vi "Update-GUI-default-params.vi"(8 "error in":errorcluster, 10 "Data ref. in":refnum<data-value>, 11 "UI ref. in":refnum<data-value>) -> (0 "error IO":errorcluster, 2 "Data ref.":refnum<data-value>, 3 "UI ref.":refnum<data-value>)   [LabVIEW 2013, in "CameraVision.lvlib" / "CV-UI.lvclass"]
doc: "This function loads the default values for the GUI program parameters from an .xml file and writes these values to the GUI controls.\nThe file path for the GUI parameters is '<Application directory>\\Program data\\parameters-gui.xml'.\nThe default hidden parameters can be changed using the 'CV-Set-gui-parameters.vi' utility."
uses:
  CV-UI.lvclass
  Main/CV-Main.lvclass
  Parameters-gui.ctl
  Main/Configuration/Configuration-parameters-gui.ctl
  Main/Acquisition/Acquisition-parameters-gui.ctl
  Main/Acquisition/Trigger-modes.ctl
  Main/Acquisition/Exposure-modes.ctl
  Main/Storage/Storage-parameters-gui.ctl
  Main/Storage/Storage-types.ctl
  Main/Correction/Correction-parameters-gui.ctl
  Main/Correction/Smoothing.ctl
  Main/Correction/Background-correction.ctl
  Main/Analysis/Analysis-parameters-gui.ctl
  Main/Temperature/Temperature-parameters-gui.ctl
  Main/Mapping/Mapping-parameters-gui.ctl
  Main/Mapping/Mapping-characteristic.ctl
  Main/Filter/Filter-parameters-gui.ctl
  Main/Filter/Filter-settings.ctl
  Main/Filter/Filter-characteristic.ctl
  Main/Filter/Filter-apply.ctl
  CV-UI.lvclass/CV-UI.ctl
  Read Parameter refs.vi
  <vilib>/Utility/xml.llb/Read From XML File(string).vi
  Main/Filter/CV-Filter.lvclass
  Main/Mapping/CV-Mapping.lvclass
  Main/Temperature/CV-Temperature.lvclass
  Main/Analysis/CV-Analysis.lvclass
  Main/Correction/CV-Correction.lvclass
  Main/Storage/CV-Storage.lvclass
  Main/Acquisition/CV-Acquisition.lvclass
  Main/Configuration/CV-Configuration.lvclass
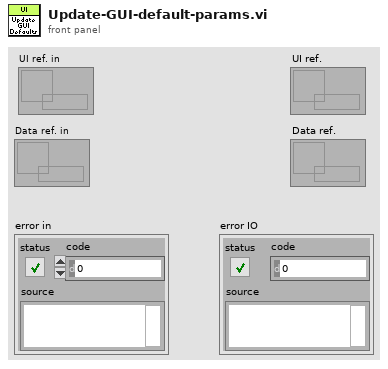
[diagram p1: front panel]
types:
  T1 = typedef "CameraVision.lvlib/CV-UI.lvclass/Parameters-gui.ctl" = cluster{"Configuration params":T2, "Acquisition params":T3, "Storage params":T6, "Correction params":T8, "Analysis params":T11, "Temperature params":T12, "Mapping params":T13, "Filter params":T15}
  T2 = typedef "CameraVision.lvlib/CV-Configuration.lvclass/Configuration-parameters-gui.ctl" = cluster{"Number of cameras":i32, "Camera 1 port":enum16{"A", "B"}, "ROI width":u32, "ROI height":u32, "Reset ROI":bool, "Width scale":dbl, "Height scale":dbl, "Center Y cam. 1":i32, "Center X cam. 1":i32, "Center Y cam. 2":i32, "Center X cam. 2":i32}
  T3 = typedef "CameraVision.lvlib/CV-Acquisition.lvclass/Acquisition-parameters-gui.ctl" = cluster{"Acquisition mode":enum16{"Continuous", "Continuous batch", "Single batch", "Single batch -delayed"}, "Batch size":i32, "Image buffer size":i32, "Trigger mode":T4, "Duration HH":sgl, "Acquisition start":enum16{"Immediate", "Post-phoned"}, "Duration SS":sgl, "Duration MM":sgl, "Start time":timestamp, "Max. frame rate":dbl, "Exposure time cam. 1":dbl, "Exposure time cam. 2":dbl, "Exposure mode":T5, "Value 1":dbl, "Value 2":dbl, "Time 1":dbl, "Time 2":dbl}
  T4 = typedef "CameraVision.lvlib/CV-Acquisition.lvclass/Trigger-modes.ctl" = enum16{"Camera timed (not sync.)", "Framegrabber timed (sync.)", "Software timed (sync.)", "External timing (sync.)", "Manual (sync.)", "Gated - camera (not sync.)", "Gated - grabber (sync.)", "Gated - software (sync.)", "Gated - external (sync.)"}
  T5 = typedef "CameraVision.lvlib/CV-Acquisition.lvclass/Exposure-modes.ctl" = enum16{"Linear", "LinLog"}
  T6 = typedef "CameraVision.lvlib/CV-Storage.lvclass/Storage-parameters-gui.ctl" = cluster{"Base file name":string, "Storage directory":path, "Save what?":T7, "Image file type":enum16{"JPG", "BMP", "PNG"}, "Comments":string, "Storage mode":enum16{"1 file per layer", "1 file for all layers "}, "Start iteration/layer":u16}
  T7 = typedef "CameraVision.lvlib/CV-Storage.lvclass/Storage-types.ctl" = cluster{"Original":bool, "Corrected":bool, "Binary":bool, "Temperature":bool, "Characteristics":bool, "Mapping":bool, "TemperatureValues":bool}
  T8 = typedef "CameraVision.lvlib/CV-Correction.lvclass/Correction-parameters-gui.ctl" = cluster{"Background correction":bool, "Hot-pixel correction":bool, "Black image cam. 1":path, "Black image cam. 2":path, "Y-shift":i32, "X-shift":i32, "Correlation algorithm":enum16{"Fixed shift", "Cross-correlation", "Cross-correlation (5steps)", "Melt-pool center"}, "Noise treshold":sgl, "Smoothing algorithm":T9, "2nd image correlation":bool, "Image smoothing":bool, "Background correction method":T10}
  T9 = typedef "CameraVision.lvlib/CV-Correction.lvclass/Smoothing.ctl" = enum16{"Noise tresholding", "NT+Median filter", "NT+Gaussian filter"}
  T10 = typedef "CameraVision.lvlib/CV-Correction.lvclass/Background-correction.ctl" = enum16{"Hardware", "Software"}
  T11 = typedef "CameraVision.lvlib/CV-Analysis.lvclass/Analysis-parameters-gui.ctl" = cluster{"Binarization treshold":sgl, "Image characteristics":bool, "Melt-pool characteristics":bool}
  T12 = typedef "CameraVision.lvlib/CV-Temperature.lvclass/Temperature-parameters-gui.ctl" = cluster{"Temperature field":bool, "Ratio correction factor":dbl, "Temperature value":bool, "Y-coord.":dbl, "X-coord.":dbl, "Averaging center":enum16{"Fixed coordinates (pixel)", "Fixed coordinates (mm)", "Melt-pool center"}, "Averaging shape":enum16{"Point", "Circle", "Ellipse"}, "Minor axis":dbl, "Major axis":dbl}
  T13 = typedef "CameraVision.lvlib/CV-Mapping.lvclass/Mapping-parameters-gui.ctl" = cluster{"Enable mapping":bool, "Automatic timing":bool, "Scan pattern file":path, "Start off-set":dbl, "Default map characteristic":T14, "Default mark speed":i32, "Jump speed":i32}
  T14 = typedef "CameraVision.lvlib/CV-Mapping.lvclass/Mapping-characteristic.ctl" = enum16{"Average intensity [0-255]", "Peak intensity [0-255]", "Melt-pool size [mm²]", "Melt-pool aspect ratio []", "Melt-pool fragments []", "Average temperature [°C]", "Max. temperature [°C]", "Min. temperature [°C]", "Std. dev. temperature [°C]"}
  T15 = typedef "CameraVision.lvlib/CV-Filter.lvclass/Filter-parameters-gui.ctl" = cluster{"Filter array":T16[], "Storage filters":T18}
  T16 = typedef "CameraVision.lvlib/CV-Filter.lvclass/Filter-settings.ctl" = cluster{"Characteristic":T17, "Monitor":bool, "Min.":dbl, "Max.":dbl, "Min. Thres.":dbl, "Min. Dur.":u16, "Report":bool}
  T17 = typedef "CameraVision.lvlib/CV-Filter.lvclass/Filter-characteristic.ctl" = enum16{"Average intensity [0-255]", "Peak intensity [0-255]", "Melt-pool size [mm²]", "Melt-pool aspect ratio []", "Melt-pool fragments []", "Melt-pool position X [pixel]", "Melt-pool position Y [pixel]", "Average temperature [°C]", "Max. temperature [°C]", "Min. temperature [°C]", "Std. dev. temperature [°C]"}
  T18 = typedef "CameraVision.lvlib/CV-Filter.lvclass/Filter-apply.ctl" = cluster{"Filter images":bool, "Filter characteristics":bool, "Filter temperature":bool}
  T19 = typedef "CameraVision.lvlib/CV-UI.lvclass/Parameter-group-names.ctl" = enum16{"Configuration params", "Acquisition params", "Correction params", "Analysis params", "Temperature params", "Mapping params", "Storage params", "Filter params"}
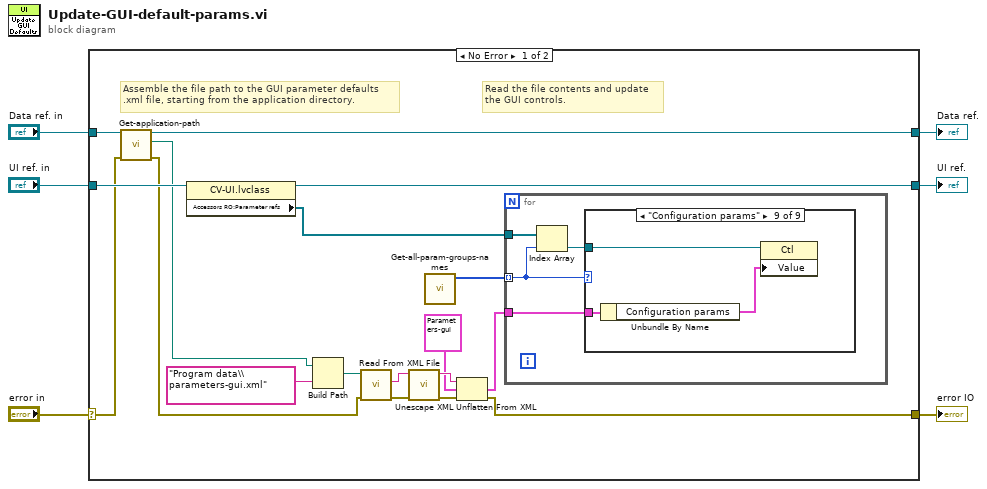
[diagram p0: block diagram]
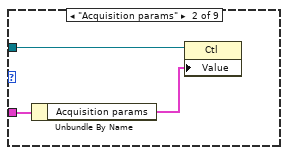
[diagram p3: hidden frame]
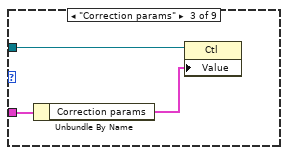
[diagram p4: hidden frame]
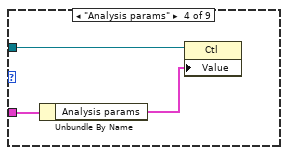
[diagram p5: hidden frame]
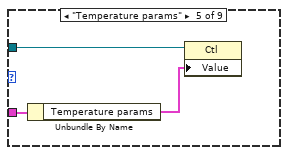
[diagram p6: hidden frame]
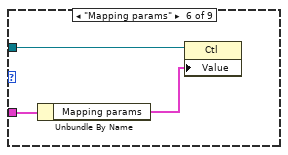
[diagram p7: hidden frame]
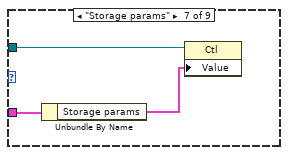
[diagram p8: hidden frame]
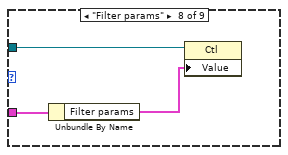
[diagram p9: hidden frame]
diagram:
  n1 = case shown="No Error" "error in" {
    selector: "error in" -> [w8 w55]
    tunnel: [w12 w55] -> w6
    tunnel: "UI ref. in" -> [w23 w54]
    tunnel: [w22 w54] -> w3
    tunnel: "Data ref. in" -> [w11 w53]
    tunnel: [w7 w53] -> w1
    frame No Error {
      # "Read the file contents and update\nthe GUI controls."
      # "Assemble the file path to the GUI parameter defaults\n.xml file, starting from the application directory."
      n2 = call "Get-application-path.vi"("error in (no error)"=w8, "Data ref. in"=w11) -> ("error out"=w9:errorcluster, "App path"=w10:path, "Data ref."=w7:refnum<data-value>)  [unwired: 7 in]
      n3 = property class="CV-UI.lvclass"(reference=w23) -> (reference out=w22:refnum<data-value>, "Accessors RO:Parameter refs"=w14:refnum<vi>[])  [unwired: 1 in, 1 out]
      n4 = Build Path(base path=w10, name or relative path="Program data\\parameters-gui.xml" ("Relative save path")) -> (appended path=w18:path)
      n5 = call-poly <vilib>:"Read From XML File.vi"("error in (no error)"=w9, "XML File Path"=w18) -> ("error out"=w17:errorcluster, "XML Elements"=w21:string)  [unwired: 7 in, 1 out]
      n6 = call <vilib>:"Unescape XML.vi"("error in (no error)"=w17, "XML String In"=w21) -> ("error out"=w16:errorcluster, "XML String Out"=w20:string)  [unwired: 8 in]
      n7 = call "Get-all-param-groups-names.vi"() -> ("Param groups"=w15:T19[])  [unwired: 11 in]
      n8 = Unflatten From XML(xml string=w20, type=T1 {"Configuration params"={"Number of cameras"=0, "Camera 1 port"=enum."B", "ROI width"=0, "ROI height"=1248, "Reset ROI"=FALSE, "Width scale"=0.0, "Height scale"=0.05, "Center Y cam. 1"=0, "Center X cam. 1"=1, "Center Y cam. 2"=1, "Center X cam. 2"=1}, "Acquisition params"={"Acquisition mode"=enum."Continuous", "Batch size"=0, "Image buffer size"=1, "Trigger mode"=enum."Camera timed (not sync.)", "Duration HH"=0.0, "Acquisition start"=enum."Post-phoned", "Duration SS"=0.01, "Duration MM"=0.01, "Start time"=timestamp(0 s since 1904-01-01), "Max. frame rate"=0.0, "Exposure time cam. 1"=0.0, "Exposure time cam. 2"=0.0, "Exposure mode"=enum."Linear", "Value 1"=0.0, "Value 2"=0.0, "Time 1"=0.0, "Time 2"=0.0}, "Storage params"={"Base file name"="", "Storage directory"=path "", "Save what?"={"Original"=FALSE, "Corrected"=FALSE, "Binary"=FALSE, "Temperature"=FALSE, "Characteristics"=FALSE, "Mapping"=FALSE, "TemperatureValues"=FALSE}, "Image file type"=enum."BMP", "Comments"="", "Storage mode"=enum."1 file per layer", "Start iteration/layer"=0}, "Correction params"={"Background correction"=FALSE, "Hot-pixel correction"=FALSE, "Black image cam. 1"=path "", "Black image cam. 2"=path "", "Y-shift"=0, "X-shift"=0, "Correlation algorithm"=enum."Fixed shift", "Noise treshold"=0.0, "Smoothing algorithm"=enum."Noise tresholding", "2nd image correlation"=FALSE, "Image smoothing"=FALSE, "Background correction method"=enum."Hardware"}, "Analysis params"={"Binarization treshold"=0.0, "Image characteristics"=FALSE, "Melt-pool characteristics"=FALSE}, "Temperature params"={"Temperature field"=FALSE, "Ratio correction factor"=0.0, "Temperature value"=FALSE, "Y-coord."=0.0, "X-coord."=0.0, "Averaging center"=enum."Fixed coordinates (pixel)", "Averaging shape"=enum."Point", "Minor axis"=0.0, "Major axis"=0.0}, "Mapping params"={"Enable mapping"=FALSE, "Automatic timing"=FALSE, "Scan pattern file"=path "", "Start off-set"=40.0, "Default map characteristic"=enum."Average intensity [0-255]", "Default mark speed"=0, "Jump speed"=0}, "Filter params"={"Filter array"=[], "Storage filters"={"Filter images"=FALSE, "Filter characteristics"=FALSE, "Filter temperature"=FALSE}}} ("Parameters"), error in (no error)=w16) -> (value=w13:T1, error out=w12:errorcluster)
      n9 = for {
        tunnel: w15 -> [w26] mode=indexing
        tunnel: w14 -> [w28]
        tunnel: w13 -> [w25]
        n10 = Index Array(array=w28, index=w26) -> (element=w27:refnum<vi>)
        n11 = case shown="\"Configuration params\"" w26 {
          tunnel: w27 -> [_ w30 w33 w36 w39 w42 w45 w48 w51]
          tunnel: w25 -> [_ w31 w34 w37 w40 w43 w46 w49 w52]
          frame Default {
          }
          frame "Acquisition params" {
            n12 = Unbundle By Name(w31) -> ("Acquisition params"=w29:T3)
            n13 = property class="Ctl"(reference=w30, "Value"=w29) -> ()  [unwired: 1 in, 2 out]
          }
          frame "Correction params" {
            n14 = Unbundle By Name(w34) -> ("Correction params"=w32:T8)
            n15 = property class="Ctl"(reference=w33, "Value"=w32) -> ()  [unwired: 1 in, 2 out]
          }
          frame "Analysis params" {
            n16 = Unbundle By Name(w37) -> ("Analysis params"=w35:T11)
            n17 = property class="Ctl"(reference=w36, "Value"=w35) -> ()  [unwired: 1 in, 2 out]
          }
          frame "Temperature params" {
            n18 = Unbundle By Name(w40) -> ("Temperature params"=w38:T12)
            n19 = property class="Ctl"(reference=w39, "Value"=w38) -> ()  [unwired: 1 in, 2 out]
          }
          frame "Mapping params" {
            n20 = Unbundle By Name(w43) -> ("Mapping params"=w41:T13)
            n21 = property class="Ctl"(reference=w42, "Value"=w41) -> ()  [unwired: 1 in, 2 out]
          }
          frame "Storage params" {
            n22 = Unbundle By Name(w46) -> ("Storage params"=w44:T6)
            n23 = property class="Ctl"(reference=w45, "Value"=w44) -> ()  [unwired: 1 in, 2 out]
          }
          frame "Filter params" {
            n24 = Unbundle By Name(w49) -> ("Filter params"=w47:T15)
            n25 = property class="Ctl"(reference=w48, "Value"=w47) -> ()  [unwired: 1 in, 2 out]
          }
          frame "Configuration params" {
            n26 = Unbundle By Name(w52) -> ("Configuration params"=w50:T2)
            n27 = property class="Ctl"(reference=w51, "Value"=w50) -> ()  [unwired: 1 in, 2 out]
          }
        }
      }
    }
    frame Error {
    }
  }
  "error IO" <- w6
  "UI ref." <- w3
  "Data ref." <- w1
